vi "receive_next_packet.vi"(2 "error in (no error)":errorcluster, 3 "timeout":u32) -> (0 "error out":errorcluster, 1 "packet":T1)   [LabVIEW 2016]
uses:
  <vilib>/SmarAct/MCS/Types/mcsPacket.ctl
  sa commands.ctl
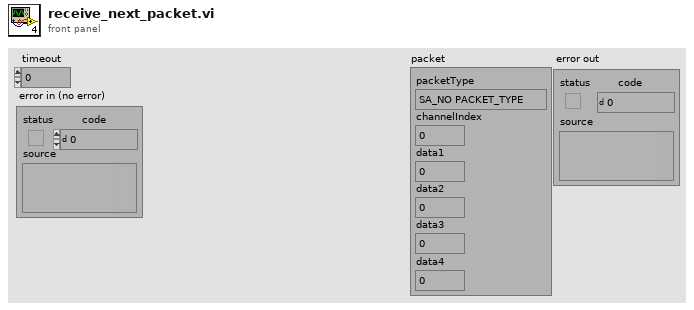
[diagram p1: front panel]
types:
  T1 = typedef "mcsPacket.ctl" = cluster{"packetType":enum32{"SA_NO PACKET_TYPE", "SA_ERROR_ PACKET_TYPE", "SA_POSITION PACKET_TYPE", "SA_COMPLETED PACKET_TYPE", "SA_STATUS PACKET_TYPE", "SA_ANGLE_PACKET_TYPE", "SA_VOLTAGE_LEVEL_PACKET_TYPE", "SA_SENSOR_TYPE_PACKET_TYPE", "SA_SENSOR_ENABLED_PACKET_TYPE", "SA_END_EFFECTOR_TYPE_PACKET_TYPE", "SA_GRIPPER_OPENING_PACKET_TYPE", "SA_FORCE_PACKET_TYPE", "SA_MOVE_SPEED_PACKET_TYPE", "SA_PHYSICAL_POSITION_KNOWN_PACKET_TYPE", "SA_POSITION_LIMIT_PACKET_TYPE", "SA_ANGLE_LIMIT_PACKET_TYPE", "SA_SAFE_DIRECTION_PACKET_TYPE", "SA_SCALE_PACKET_TYPE", "SA_MOVE_ACCELERATION_PACKET_TYPE", "SA_CHANNEL_PROPERTY_PACKET_TYPE", "SA_CAPTURE_BUFFER_PACKET_TYPE", "SA_TRIGGERED_PACKET_TYPE"}, "channelIndex":u32, "data1":u32, "data2":i32, "data3":i32, "data4":u32}
  T2 = typedef "sa commands.ctl" = enum16{"read all", "set system index", "set x channel", "set y channel", "set rotation channel"}
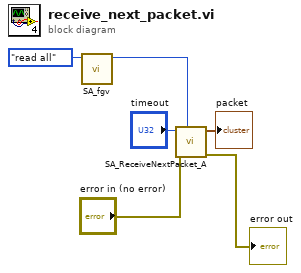
[diagram p0: block diagram]
diagram:
  n1 = call "SA_fgv.vi"("command"=sa_commands."read all") -> ("system index"=w6:u32)  [unwired: 3 in, 3 out]
  n2 = call <vilib>:"SA_ReceiveNextPacket_A.vi"("systemIndex"=w6, "error in (no error)"="error in (no error)", "timeout"="timeout") -> ("error out"=→"error out":errorcluster, "packet"=→"packet":T1)  [unwired: 7 in]
